vi "Produce AO.vi"(9 "SW Signal":i16, 10 "Cell 1":T1 {"f0" format="%.32g"; "Scale" format="%.14g"}) -> (3 "AO":i16)   [LabVIEW 2018]
uses:
  <vilib>/rvi/FXPMathLib/FxpMul/XNode/nifxpmath_Multiplier.xnode
  <vilib>/rvi/FXPMathLib/FxpAdd/XNode/nifxpmath_Add.xnode
  <vilib>/rvi/FXPMathLib/sim/FxpSim.dll
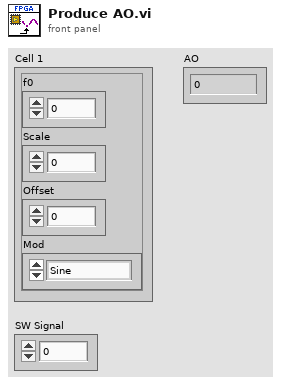
[diagram p1: front panel]
types:
  T1 = cluster{"f0":fxp<+,32,0>, "Scale":fxp<+,14,1>, "Offset":i16, "Mod":enum8{"Sine", "Square"}}
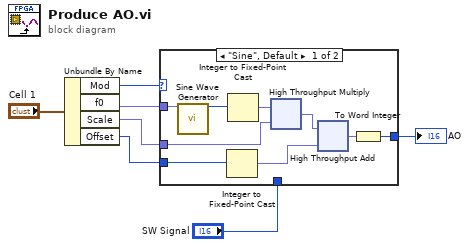
[diagram p0: block diagram]
diagram:
  n1 = Unbundle By Name("Cell 1") -> ("Mod"=w3:enum8{"Sine", "Square"}, "f0"=w4:fxp<+,32,0>, "Scale"=w5:fxp<+,14,1>, "Offset"=w6:i16)
  n2 = case shown="\"Sine\", Default" w3 {
    tunnel: w6 -> [w16 _]
    tunnel: w5 -> [w15 _]
    tunnel: w4 -> [w14 _]
    tunnel: [w8 w17] -> w2
    tunnel: "SW Signal" -> [_ w17]
    frame "Sine", Default {
      n3 = call "Sine Wave Generator"("frequency (periods/tick)"=w14) -> ("sine out"=w11:i16)  [unwired: 14 in]
      n4 = Integer to Fixed-Point Cast(integer=w16) -> (fixed-point=w13:fxp<+/-,16,16>)  [unwired: 1 in]
      n5 = Integer to Fixed-Point Cast(integer=w11) -> (fixed-point=w12:fxp<+/-,16,16>)  [unwired: 1 in]
      n6 = xnode ("High Throughput Multiply")("x"=w12, "y"=w15) -> ("x*y"=w9:fxp<+/-,16,16>)
      n7 = xnode ("High Throughput Add")("x"=w9, "y"=w13) -> ("x+y"=w10:fxp<+/-,16,16>)
      n8 = To Word Integer(number=w10) -> (16bit integer=w8:i16)
    }
    frame "Square" {
    }
  }
  "AO" <- w2
